vi "get index type definitions.vi"(10 "channel classification":T1, 11 "System Diagnostics configuration in":refnum<class "System Diagnostics configuration.lvclass">) -> (1 "valid?":bool, 2 "index cluster":variant, 3 "System Diagnostics configuration out":refnum<class "System Diagnostics configuration.lvclass">)   [LabVIEW 2013, in "System Diagnostics configuration.lvclass"]
uses:
  System Diagnostics configuration.lvclass
  <vilib>/NI/Tag Bus Module Framework/channel/channel classification.ctl
  input data indices.ctl
  <vilib>/NI/Tag Bus Module Framework/channel/TBM channel.lvclass
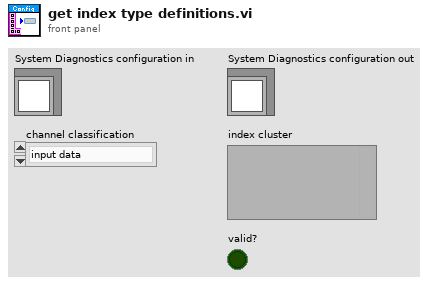
[diagram p1: front panel]
types:
  T1 = typedef "TBM channel.lvclass/channel classification.ctl" = enum16{"input data", "output data", "processing parameter", "processing result"}
  T2 = typedef "System Diagnostics configuration.lvclass/input data indices.ctl" = cluster{"Double.CPU load average":i32, "Double.timed structures load":i32, "Double.free memory":i32, "Double.contiguous memory":i32}
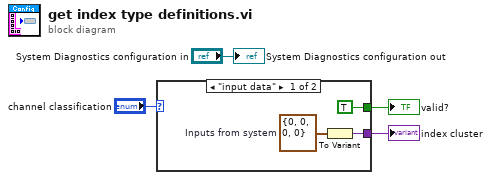
[diagram p0: block diagram]
diagram:
  n1 = case shown="\"input data\"" "channel classification" {
    tunnel: [TRUE _] -> w2
    tunnel: [w5 _] -> w1
    frame "input data" {
      w6 = T2 {"Double.CPU load average"=0, "Double.timed structures load"=0, "Double.free memory"=0, "Double.contiguous memory"=0}  # Inputs from system
      n2 = To Variant(anything=w6) -> (Variant=w5:variant)
    }
    frame Default {
    }
  }
  "valid?" <- w2
  "index cluster" <- w1
  "System Diagnostics configuration out" <- "System Diagnostics configuration in"
